vi "Battery Voltage.vi"(8 "error in (no error)":errorcluster, 11 "VISA resource name":refnum<visa-resource-name>) -> (0 "error out":errorcluster, 2 "Battery Voltage":dbl format="%#.2f", 3 "VISA resource name out":refnum<visa-resource-name>)   [LabVIEW 2015, in "Keysight U1252.lvlib"]
doc: "This VI gets Battery voltage inside instrument."
uses:
  <instrlib>/Keysight U1252/Keysight U1252.lvlib
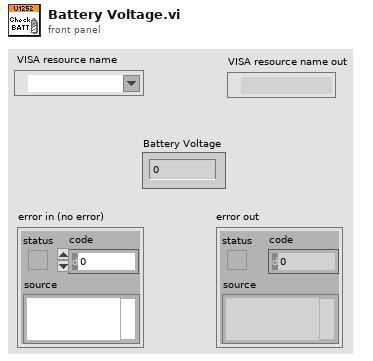
[diagram p1: front panel]
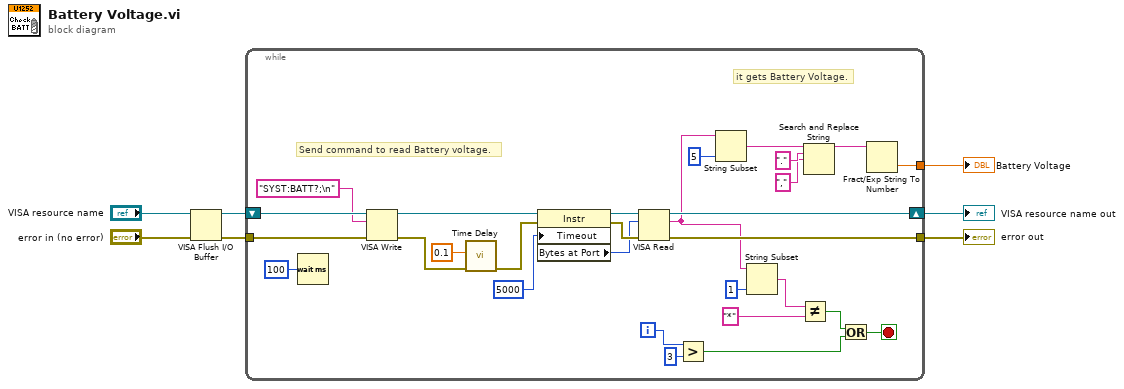
[diagram p0: block diagram]
diagram:
  n1 = VISA Flush I/O Buffer(VISA resource name="VISA resource name", error in (no error)="error in (no error)") -> (VISA resource name out=w2:refnum<visa-resource-name>, error out=w3:errorcluster)  [unwired: 1 in]
  n2 = while {
    shift-right: [w35] -> w6
    shift-left: w2 -> [w36]
    tunnel: w3 -> [w27]
    tunnel: [w24] -> w7
    tunnel: [w14] -> w1
    i -> [w29]
    stop <- w16 stop-if-true
    # "it gets Battery Voltage."
    # "Send command to read Battery voltage."
    n3 = Wait (ms)(milliseconds to wait=u32 100) -> ()  [unwired: 1 out]
    n4 = VISA Write(VISA resource name=w36, write buffer="SYST:BATT?;\n", error in (no error)=w27) -> (VISA resource name out=w33:refnum<visa-resource-name>, error out=w19:errorcluster)  [unwired: 1 out]
    n5 = call "Time Delay"("error in (no error)"=w19, "Delay Time (s)"=0.1) -> ("error out"=w18:errorcluster)  [unwired: 9 in]
    n6 = property class="Instr"(reference=w33, error in=w18, "Timeout"=u32 5000 ("General Settings:Timeout Value")) -> (reference out=w31:refnum<visa-resource-name>, error out=w30:errorcluster, "Bytes at Port"=w21:u32)
    n7 = VISA Read(VISA resource name=w31, byte count=w21, error in (no error)=w30) -> (VISA resource name out=w35:refnum<visa-resource-name>, read buffer=w10:string, error out=w24:errorcluster)  [unwired: 1 out]
    n8 = Greater?(x=w29, y=3) -> (0:w15:bool)
    n9 = String Subset(string=w10, length (rest)=5 ("length (rest)")) -> (substring=w8:string)  [unwired: 1 in]
    n10 = String Subset(string=w10, length (rest)=1 ("length (rest)")) -> (substring=w22:string)  [unwired: 1 in]
    n11 = Not Equal?(x=w22, y="*") -> (x != y?=w17:bool)
    n12 = Search and Replace String(input string=w8, search string=".", replace string="," ("replace string (\"\")")) -> (result string=w11:string)  [unwired: 5 in, 3 out]
    n13 = Or(x=w17, y=w15) -> (x .or. y?=w16:bool)
    n14 = Fract/Exp String To Number(string=w11) -> (number=w14:dbl)  [unwired: 3 in, 1 out]
  }
  "error out" <- w7
  "VISA resource name out" <- w6
  "Battery Voltage" <- w1
